vi "调用库函数截图.vi"() -> ()   [LabVIEW 2014]
uses:
  <vilib>/picture/picture.llb/imagedata.ctl
  CameraDll.dll
panel:
  out "new picture":picture caption="新图片"
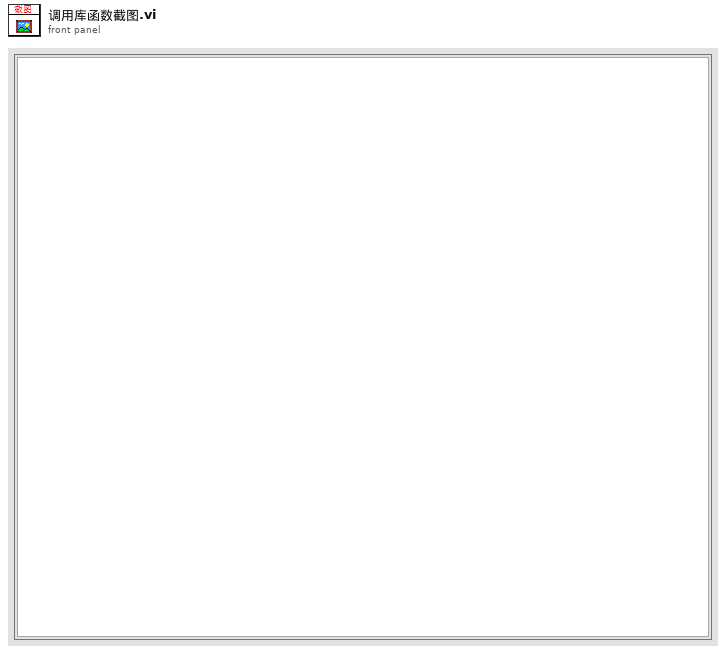
[diagram p1: front panel]
types:
  T1 = enum32{"Invalid", "Standard", "Closed", "Hidden", "Minimized", "Maximized"}
  T2 = typedef "imagedata.ctl" = cluster{"image type":i32, "image depth":i32, "image":u8[], "mask":u8[], "colors":u32[], "Rectangle":cluster{"left":i16, "top":i16, "right":i16, "bottom":i16}}
  T3 = typedef "LVRectTypeDef.ctl" = cluster{"Left":i16, "Top":i16, "Right":i16, "Bottom":i16}
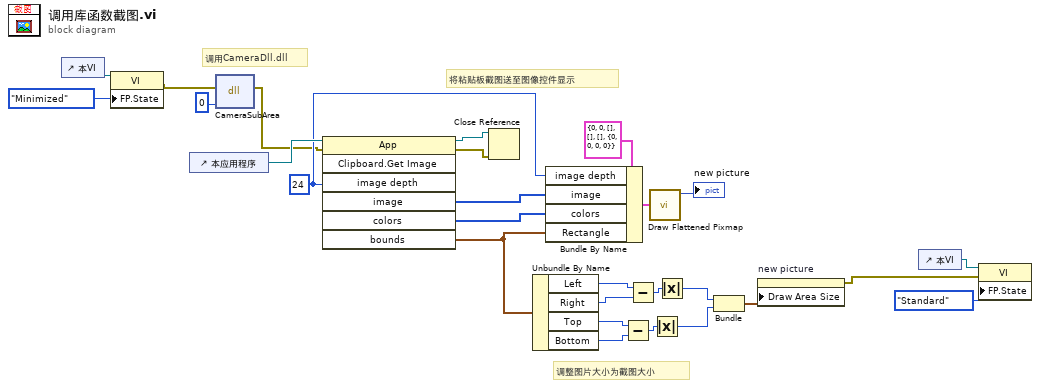
[diagram p0: block diagram]
diagram:
  w26 = 24 ("图像深度")
  # "将粘贴板截图送至图像控件显示"
  # "调用CameraDll.dll"
  # "调整图片大小为截图大小"
  n1 = control-ref of="本VI"() -> (w16:refnum<vi>)
  n2 = property class="VI"(reference=w16, "FP.State"=T1."Minimized" ("前面板窗口:状态")) -> (error out=w14:errorcluster)  [unwired: 1 in, 1 out]
  n3 = control-ref of="本应用程序"() -> (w27:refnum<vi>)
  n4 = dll-call lib="PTH2Aabs CUsersvsDesktop调用库函数截图\nCameraDll.dll" fn="CameraSubArea"(error in=w14, "int"=0) -> (error out=w18:errorcluster)  [unwired: 4 in, 1 out]
  n5 = invoke class="App" method="Clipboard.Get Image"(reference=w27, error in=w18, "image depth"=w26) -> (reference out=w20:refnum<vi>, error out=w19:errorcluster, "image"=w25:u8[], "colors"=w24:u32[], "bounds"=w11:T3)  [unwired: 4 in, 2 out]
  n6 = Close Reference(reference=w20, error in (no error)=w19) -> ()  [unwired: 1 out]
  n7 = Unbundle By Name(w11) -> ("Left"=w9:i16, "Right"=w8:i16, "Top"=w6:i16, "Bottom"=w5:i16)
  n8 = Bundle By Name(cluster=T2 {"image type"=0, "image depth"=0, "image"=[], "mask"=[], "colors"=[], "Rectangle"={"left"=0, "top"=0, "right"=0, "bottom"=0}} ("image data"), "image depth"=w26, "image"=w25, "colors"=w24, "Rectangle"=w11) -> (w22:T2)
  n9 = Subtract(x=w6, y=w5) -> (x-y=w7:i16)
  n10 = Subtract(x=w9, y=w8) -> (x-y=w10:i16)
  n11 = call <vilib>:"Draw Flattened Pixmap.vi"("image data"=w22) -> ("new picture"=→"new picture":picture)  [unwired: 8 in]
  n12 = Absolute Value(x=w7) -> (abs(x)=w3:i16)
  n13 = Absolute Value(x=w10) -> (abs(x)=w4:i16)
  n14 = Bundle(w4, w3) -> (w2:cluster{i16, i16})  [unwired: 1 in]
  n15 = property on="new picture" class="Pict"("Draw Area Size"=w2) -> (error out=w1:errorcluster)  [unwired: 2 in, 1 out]
  n16 = control-ref of="本VI"() -> (w12:refnum<vi>)
  n17 = property class="VI"(reference=w12, error in=w1, "FP.State"=T1."Standard" ("前面板窗口:状态")) -> ()  [unwired: 2 out]
